vi "SQL_test_template_find_testName.vi"(11 "模板名称":string) -> (3 "模板是否存在":bool)   [LabVIEW 2014]
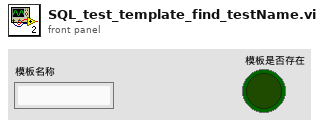
[diagram p1: front panel]
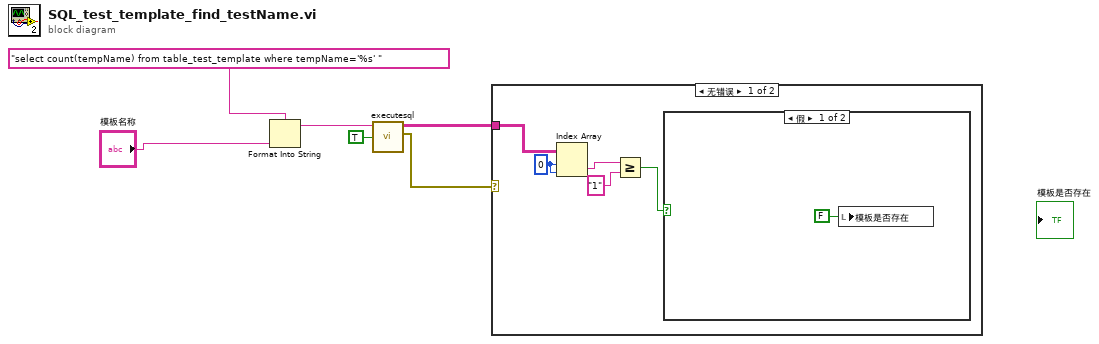
[diagram p0: block diagram]
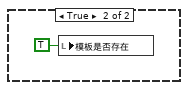
[diagram p2: hidden frame]
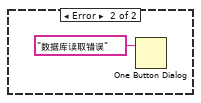
[diagram p3: hidden frame]
diagram:
  n1 = Format Into String(format string="select count(tempName) from table_test_template where tempName='%s' ", "模板名称") -> (resulting string=w5:string)  [unwired: 2 in, 1 out]
  n2 = call "executesql.vi"("Return Data (T)"=TRUE, "Command Text"=w5) -> ("error out"=w3:errorcluster, "Data"=w2:string[][])  [unwired: 5 in]
  n3 = case shown="无错误" w3 {
    tunnel: w2 -> [w8 _]
    frame No Error {
      w11 = 0 ("索引 (行)")
      n4 = Index Array(array=w8, index (row)=w11, index (col)=w11) -> (element=w10:string)
      n5 = Greater Or Equal?(x=w10, y="1") -> (x >= y?=w7:bool)
      n6 = case shown="假" w7 {
        frame False {
          n7 = local write "模板是否存在"(FALSE ("模板是否存在")) -> ()
        }
        frame True {
          n8 = local write "模板是否存在"(TRUE ("模板是否存在")) -> ()
        }
      }
    }
    frame Error {
      n9 = One Button Dialog(message="数据库读取错误" ("消息")) -> ()  [unwired: 1 in, 1 out]
    }
  }
